vi "luz_graph.vi"(11 "file path (dialog if empty)":path) -> (3 "Curva de luz":cluster{"Ramp Pattern":dbl[], u32[]}(graph))   [LabVIEW 2021]
uses:
  <vilib>/Analysis/1siggen.llb/Ramp Pattern by Delta.vi
  <vilib>/Analysis/NI_AALBase.lvlib
panel:
  in  "Filtro?":bool
  in  "True pares":bool
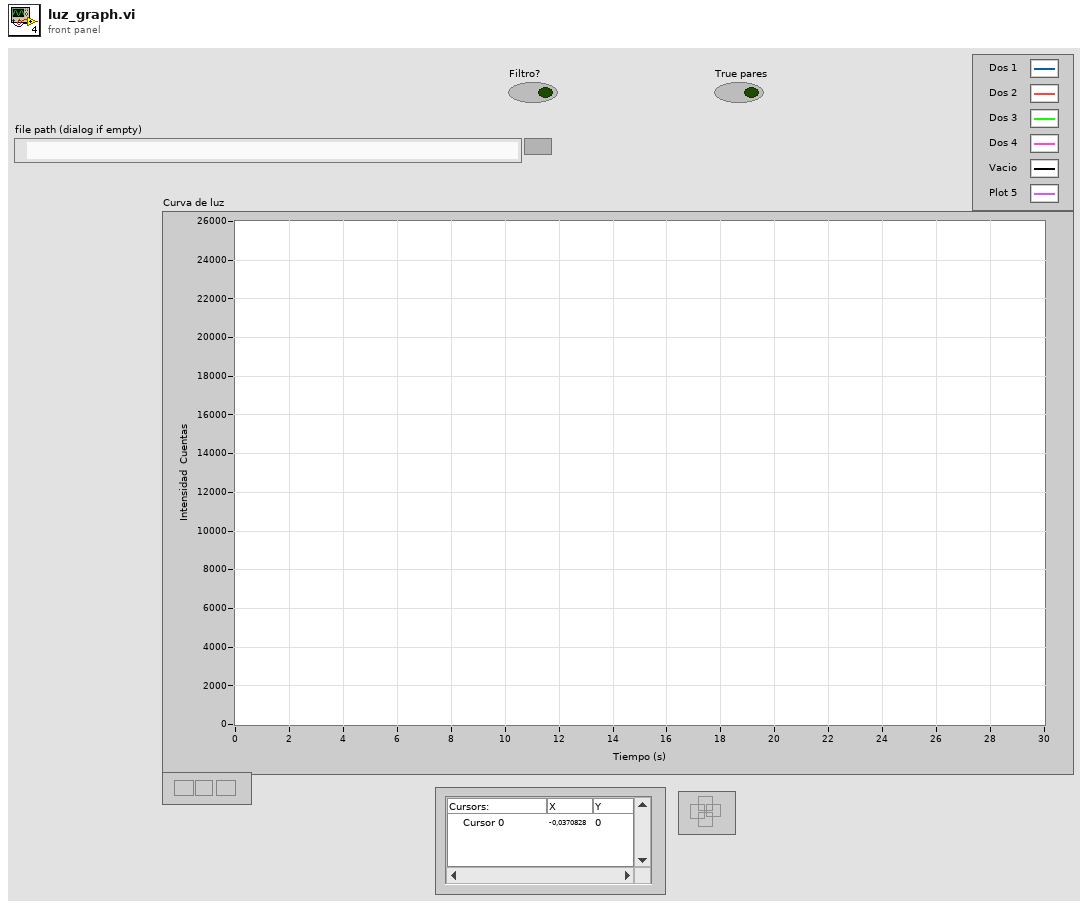
[diagram p1: front panel]
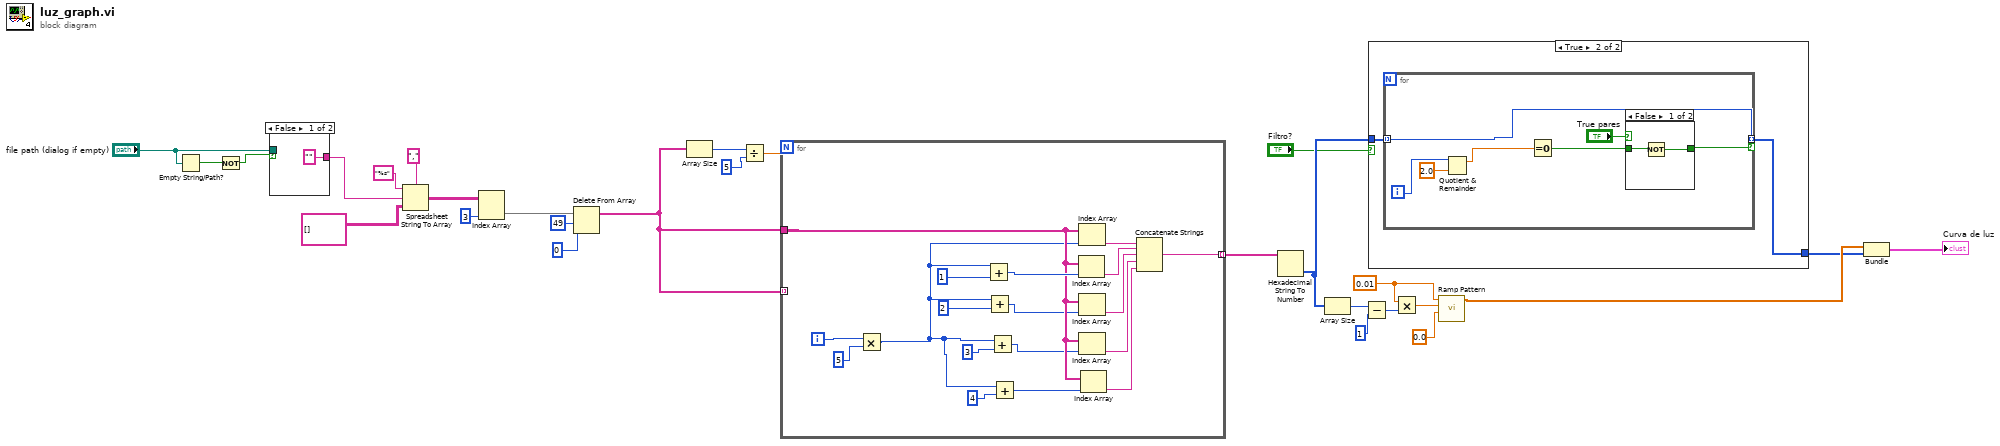
[diagram p0: block diagram]
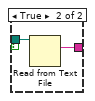
[diagram p2: hidden frame]
diagram:
  w8 = 0.01 ("delta")
  n1 = Empty String/Path?(string/path="file path (dialog if empty)") -> (empty?=w2:bool)
  n2 = Not(x=w2) -> (.not. x?=w1:bool)
  n3 = case shown="False" w1 {
    tunnel: ["" w31] -> w14
    tunnel: "file path (dialog if empty)" -> [_ w30]
    frame False {
    }
    frame True {
      n4 = Read from Text File(file (use dialog)=w30) -> (text=w31:string)  [unwired: 3 in, 3 out]
    }
  }
  n5 = Spreadsheet String To Array(delimiter (Tab)=",", format string="%s", spreadsheet string=w14, array type (2D Dbl)=string[][] [] ("Array")) -> (array=w17:string[][])
  n6 = Index Array(array=w17, index (col)=3 ("disabled index (col)")) -> (element=w19:string[])  [unwired: 1 in]
  n7 = Delete From Array(array=w19, length=49, index=0) -> (array with subset deleted=w22:string[])  [unwired: 1 out]
  n8 = Array Size(array=w22) -> (size(s)=w23:i32)
  n9 = Divide(x=w23, y=5) -> (x/y=w25:dbl)
  n10 = for {
    N: w25 -> [_]
    tunnel: w22 -> [_] mode=indexing
    tunnel: w22 -> [w40]
    tunnel: [w46] -> w26 mode=indexing
    i -> [w42]
    n11 = Multiply(x=w42, y=5) -> (x*y=w34:i32)
    n12 = Add(x=w34, y=1) -> (x+y=w43:i32)
    n13 = Add(x=w34, y=2) -> (x+y=w39:i32)
    n14 = Add(x=w34, y=3) -> (x+y=w38:i32)
    n15 = Add(x=w34, y=4) -> (x+y=w36:i32)
    n16 = Index Array(array=w40, index=w43) -> (element=w48:string)
    n17 = Index Array(array=w40, index=w34) -> (element=w49:string)
    n18 = Index Array(array=w40, index=w39) -> (element=w47:string)
    n19 = Index Array(array=w40, index=w38) -> (element=w33:string)
    n20 = Index Array(array=w40, index=w36) -> (element=w32:string)
    n21 = Concatenate Strings(w49, w48, w47, w33, w32) -> (w46:string)
  }
  n22 = Hexadecimal String To Number(string=w26) -> (number=w12:u32[])  [unwired: 2 in, 1 out]
  n23 = Array Size(array=w12) -> (size(s)=w6:i32)
  n24 = Subtract(x=w6, y=1) -> (x-y=w4:i32)
  n25 = case shown="True" "Filtro?" {
    tunnel: w12 -> [w50 w52]
    tunnel: [w50 w51] -> w11
    frame False {
    }
    frame True {
      n26 = for {
        tunnel: w52 -> [w56] mode=indexing
        tunnel: [w56] -> w51 mode=indexing if=w53
        i -> [w58]
        n27 = Quotient & Remainder(x=w58, y=2.0) -> (x-y*floor(x/y)=w57:dbl)  [unwired: 1 out]
        n28 = Equal To 0?(x=w57) -> (x = 0?=w54:bool)
        n29 = case shown="False" "True pares" {
          tunnel: w54 -> [w61 w62]
          tunnel: [w60 w62] -> w53
          frame False {
            n30 = Not(x=w61) -> (.not. x?=w60:bool)
          }
          frame True {
          }
        }
      }
    }
  }
  n31 = Multiply(x=w8, y=w4) -> (x*y=w7:dbl)
  n32 = call-poly <vilib>:"Ramp Pattern.vi"("start"=0.0, "end"=w7, "delta"=w8) -> ("Ramp Pattern"=w28:dbl[])  [unwired: 6 in, 2 out]
  n33 = Bundle("Ramp Pattern"=w28, w11) -> (→"Curva de luz":cluster{"Ramp Pattern":dbl[], u32[]})  [unwired: 1 in]
